vi "FPGA_DAC_move.vi"   [LabVIEW 2010]
uses:
  <vilib>/rvi/DataTransferAndStorage/Container/XNode/niFpgaContainer.xnode
  <vilib>/eio/EIONode/EIONode.xnode
  <vilib>/rvi/eio/nirviEIOImplementation/nirviEIOImplementation.xnode
  <vilib>/rvi/eio/common/nirviEmuClasses.ctl
  <vilib>/rvi/FIFO/Fifo_Resource/nirvififoEmulationSetSize.vi
  <vilib>/rvi/DataTransferAndStorage/Container/Common/niFpgaContainerGetUniqueNameForEmu.vi
  <vilib>/rvi/eio/common/nirviEmuTemplateMethod_noerrors.vi
types:
  T1 = typedef "nirviEmuClasses.ctl" = enum16{"IO Read", "IO Write", "Method", "Property Read", "Property Write"}
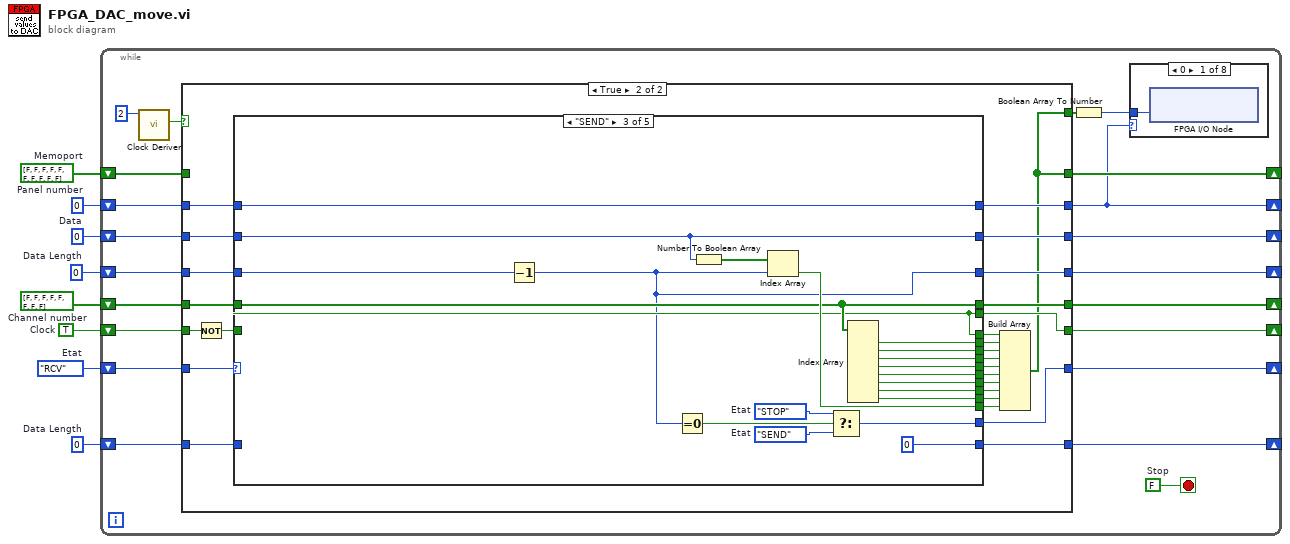
[diagram p0: block diagram]
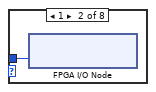
[diagram p2: hidden frame]
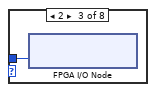
[diagram p3: hidden frame]
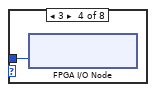
[diagram p4: hidden frame]
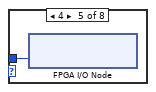
[diagram p5: hidden frame]
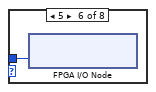
[diagram p6: hidden frame]
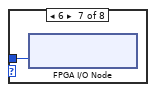
[diagram p7: hidden frame]
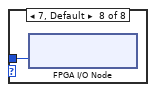
[diagram p8: hidden frame]
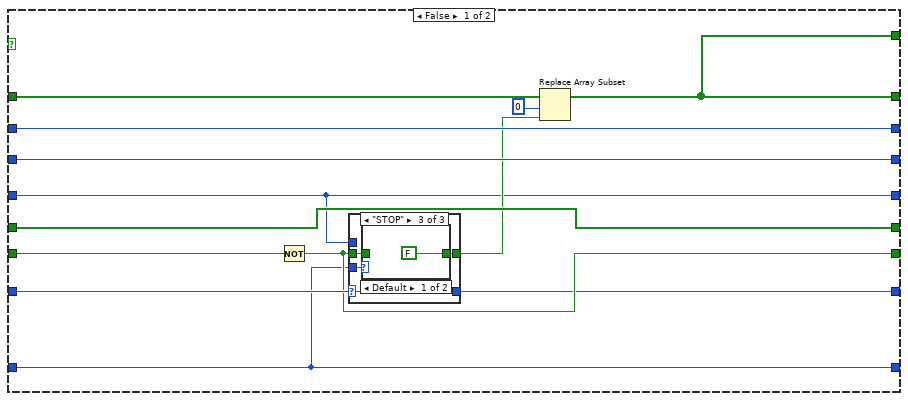
[diagram p9: hidden frame]
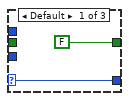
[diagram p10: hidden frame]
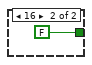
[diagram p12: hidden frame]
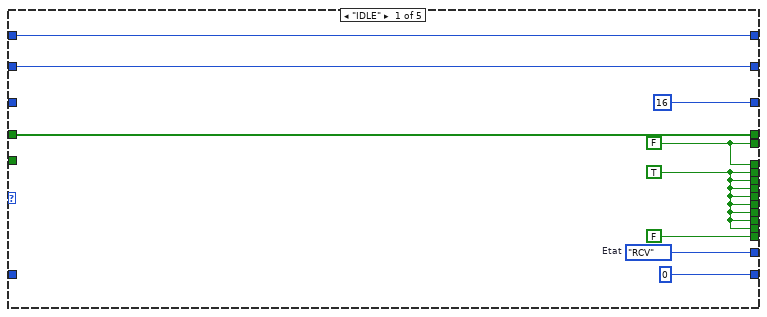
[diagram p14: hidden frame]
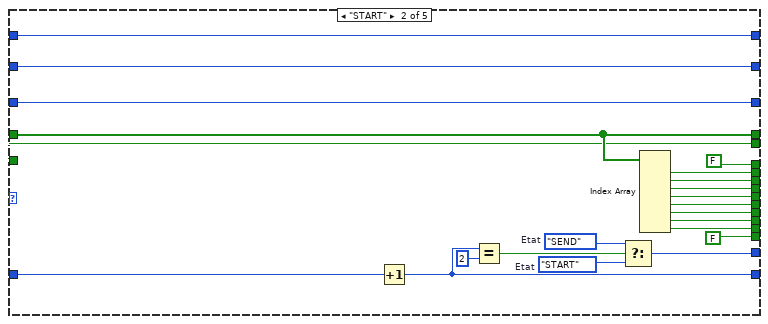
[diagram p15: hidden frame]
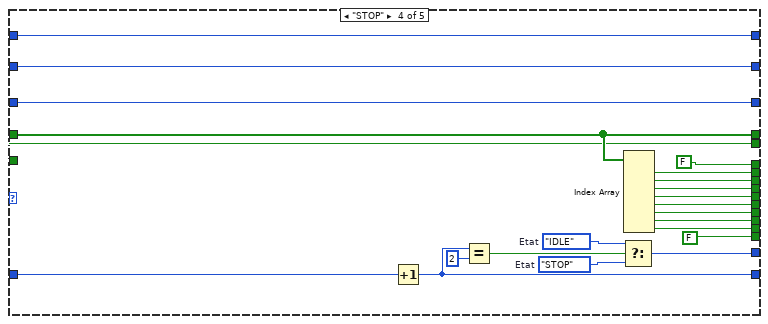
[diagram p16: hidden frame]
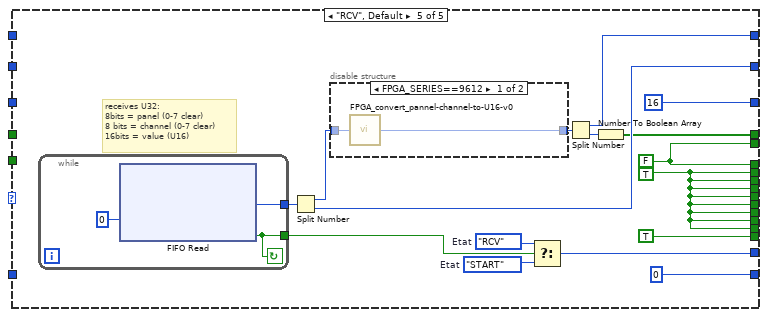
[diagram p17: hidden frame]
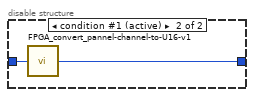
[diagram p18: hidden frame]
diagram:
  w1 = enum8{"IDLE", "START", "SEND", "STOP", "RCV"}."RCV"  # Etat
  w8 = u8 0  # Panel number
  w7 = bool[] [FALSE, FALSE, FALSE, FALSE, FALSE, FALSE, FALSE, FALSE]  # Channel number
  w6 = bool[] [FALSE, FALSE, FALSE, FALSE, FALSE, FALSE, FALSE, FALSE, FALSE, FALSE]  # Memoport
  w5 = u8 0  # Data Length
  w4 = 0  # Data Length
  w3 = u16 0  # Data
  w2 = TRUE  # Clock
  n1 = while {
    shift-right: [w23] -> _
    shift-left: w2 -> [w20]
    shift-right: [w29] -> _
    shift-left: w1 -> [w10]
    shift-right: [w28] -> _
    shift-left: w3 -> [w25]
    shift-right: [w27] -> _
    shift-left: w4 -> [w26]
    shift-right: [w22] -> _
    shift-left: w5 -> [w24]
    shift-right: [w19] -> _
    shift-left: w6 -> [w18]
    shift-right: [w17] -> _
    shift-left: w7 -> [w16]
    shift-right: [w13] -> _
    shift-left: w8 -> [w14]
    stop <- w9 stop-if-true
    w9 = FALSE  # Stop
    n2 = call "Clock Deriver.vi"("Divisor"=u32 2) -> ("Clock Out"=w21:bool)  [unwired: 1 in, 9 out]
    n3 = case shown="True" w21 {
      tunnel: w10 -> [w131 w178]
      tunnel: [w126 w177] -> w29
      tunnel: [w138 w176] -> w28
      tunnel: [w127 w175] -> w27
      tunnel: w26 -> [w127 w174]
      tunnel: w25 -> [w138 w173]
      tunnel: w20 -> [w134 w157]
      tunnel: w24 -> [w128 w172]
      tunnel: [w130 w156] -> w23
      tunnel: [w128 w171] -> w22
      tunnel: [w132 w154] -> w19
      tunnel: w18 -> [w137 _]
      tunnel: [w135 w162] -> w17
      tunnel: w16 -> [w135 w161]
      tunnel: [w133 w159] -> w13
      tunnel: w14 -> [w133 w160]
      tunnel: [w132 w154] -> w11
      frame False {
        n4 = Not(x=w134) -> (.not. x?=w130:bool)
        n5 = case shown="\"STOP\"" w131 {
          selector: w131 -> [w139 w141 w147]
          tunnel: w130 -> [_ w144 w149]
          tunnel: [FALSE w143 w148] -> w129
          tunnel: w128 -> [_ _ w150]
          tunnel: w127 -> [_ w142 _]
          tunnel: [w139 w141 w147] -> w126
          frame Default {
          }
          frame "SEND" {
            n6 = case shown="Default" w142 {
              tunnel: w144 -> [w145 _]
              tunnel: [w145 FALSE] -> w143
              frame Default {
              }
              frame 16 {
              }
            }
          }
          frame "STOP" {
            n7 = case shown="Default" w150 {
              tunnel: w149 -> [_ w152]
              tunnel: [FALSE w152] -> w148
              frame Default {
              }
              frame 0 {
              }
            }
          }
        }
        n8 = Replace Array Subset(array=w137, new element=w129, index=0) -> (w132:bool[])
      }
      frame True {
        n9 = Not(x=w157) -> (.not. x?=w155:bool)
        n10 = case shown="\"SEND\"" w178 {
          tunnel: [w180 w205 w225 w248 w263] -> w177
          tunnel: [w185 w202 w222 w245 w268] -> w164
          tunnel: [w185 w201 w221 w244 w268] -> w165
          tunnel: [w185 w200 w220 w243 w268] -> w166
          tunnel: [w185 w198 w218 w241 w268] -> w168
          tunnel: [w185 w197 w217 w240 w268] -> w169
          tunnel: [w185 w196 w216 w239 w268] -> w170
          tunnel: [FALSE ("CS") FALSE ("CS") w229 FALSE ("CS") TRUE ("CS")] -> w158
          tunnel: [w185 w199 w219 w242 w268] -> w167
          tunnel: [w181 w209 w227 w251 w265] -> w176
          tunnel: [16 ("Data Length") w208 w212 w250 16 ("Data Length")] -> w175
          tunnel: w174 -> [_ w208 w228 w250 _]
          tunnel: w173 -> [w181 w209 w227 w251 _]
          tunnel: w155 -> [_ w193 w213 w236 _]
          tunnel: w172 -> [_ w204 _ w249 _]
          tunnel: [w179 w193 w213 w236 w253] -> w156
          tunnel: [u8 0 ("Data Length") w189 u8 0 ("Data Length") w232 u8 0 ("Data Length")] -> w171
          tunnel: [w185 w203 w223 w246 w268] -> w163
          tunnel: [w183 w195 w215 w238 w264] -> w162
          tunnel: w161 -> [w183 w195 w215 w238 _]
          tunnel: [w182 w194 w214 w237 w255] -> w159
          tunnel: w160 -> [w182 w194 w214 w237 _]
          tunnel: [w179 FALSE w213 FALSE w253] -> w153
          frame "IDLE" {
            w180 = enum8{"IDLE", "START", "SEND", "STOP", "RCV"}."RCV"  # Etat
            w179 = FALSE
            w185 = TRUE ("CS")
          }
          frame "START" {
            w190 = enum8{"IDLE", "START", "SEND", "STOP", "RCV"}."START"  # Etat
            w191 = enum8{"IDLE", "START", "SEND", "STOP", "RCV"}."SEND"  # Etat
            n11 = Increment(x=w204) -> (x+1=w189:u8)
            n12 = Equal?(x=w189, y=u8 2) -> (x = y?=w206:bool)
            n13 = Select(t=w191, s=w206, f=w190) -> (s? t:f=w205:enum8{"IDLE", "START", "SEND", "STOP", "RCV"})
            n14 = Index Array(array=w195) -> (element #1=w203:bool, element #2=w202:bool, element #3=w201:bool, element #4=w200:bool, element #5=w199:bool, element #6=w198:bool, element #7=w197:bool, element #8=w196:bool)  [unwired: 8 in]
          }
          frame "SEND" {
            w210 = enum8{"IDLE", "START", "SEND", "STOP", "RCV"}."SEND"  # Etat
            w211 = enum8{"IDLE", "START", "SEND", "STOP", "RCV"}."STOP"  # Etat
            n15 = Decrement(x=w228) -> (x-1=w212:i32)
            n16 = Equal To 0?(x=w212) -> (x = 0?=w226:bool)
            n17 = Number To Boolean Array(number=w227) -> (Boolean array=w230:bool[])
            n18 = Index Array(array=w230, index=w212) -> (element=w229:bool)
            n19 = Select(t=w211, s=w226, f=w210) -> (s? t:f=w225:enum8{"IDLE", "START", "SEND", "STOP", "RCV"})
            n20 = Index Array(array=w215) -> (element #1=w223:bool, element #2=w222:bool, element #3=w221:bool, element #4=w220:bool, element #5=w219:bool, element #6=w218:bool, element #7=w217:bool, element #8=w216:bool)  [unwired: 8 in]
          }
          frame "STOP" {
            w233 = enum8{"IDLE", "START", "SEND", "STOP", "RCV"}."STOP"  # Etat
            w234 = enum8{"IDLE", "START", "SEND", "STOP", "RCV"}."IDLE"  # Etat
            n21 = Increment(x=w249) -> (x+1=w232:u8)
            n22 = Equal?(x=w232, y=u8 2) -> (x = y?=w247:bool)
            n23 = Select(t=w234, s=w247, f=w233) -> (s? t:f=w248:enum8{"IDLE", "START", "SEND", "STOP", "RCV"})
            n24 = Index Array(array=w238) -> (element #1=w246:bool, element #2=w245:bool, element #3=w244:bool, element #4=w243:bool, element #5=w242:bool, element #6=w241:bool, element #7=w240:bool, element #8=w239:bool)  [unwired: 8 in]
          }
          frame "RCV", Default {
            w258 = enum8{"IDLE", "START", "SEND", "STOP", "RCV"}."RCV"  # Etat
            w259 = enum8{"IDLE", "START", "SEND", "STOP", "RCV"}."START"  # Etat
            w253 = FALSE
            w268 = TRUE ("CS")
            # "receives U32:\n8bits = panel (0-7 clear)\n8 bits = channel (0-7 clear)\n16bits = value (U16)"
            n25 = while {
              tunnel: [w271] -> w261
              tunnel: [w269] -> w260
              stop <- w269 continue-if-true
              n26 = xnode ("FIFO Read")("Timeout"=0) -> ("Element"=w271:u32, "Timed Out?"=w269:bool)  [unwired: 1 in, 1 out]
            }
            n27 = Split Number(x=w261) -> (hi(x)=w257:u16, lo(x)=w265:u16)
            n28 = disable-structure shown="FPGA_SERIES==9612" {
              disable-tunnel: [w324 w325] -> w256
              disable-tunnel: w257 -> [w323 w326]
              frame condition #0 {
                n29 = call "FPGA_convert_pannel-channel-to-U16-v0.vi"("pannel|channel"=w323) -> ("Numérique"=w324:u16)
              }
              frame condition #1 (active) {
                n30 = call "FPGA_convert_pannel-channel-to-U16-v1.vi"("pannel|channel"=w326) -> ("Numérique"=w325:u16)
              }
            }
            n31 = Select(t=w258, s=w260, f=w259) -> (s? t:f=w263:enum8{"IDLE", "START", "SEND", "STOP", "RCV"})
            n32 = Split Number(x=w256) -> (hi(x)=w255:u8, lo(x)=w254:u8)
            n33 = Number To Boolean Array(number=w254) -> (Boolean array=w264:bool[])
          }
        }
        n34 = Build Array(w153, w163, w164, w165, w166, w167, w168, w169, w170, w158) -> (w154:bool[])
      }
    }
    n35 = Boolean Array To Number(Boolean array=w11) -> (number=w12:u16)
    n36 = case shown="0" w13 {
      tunnel: w12 -> [w30 w42 w54 w66 w78 w90 w102 w114]
      frame 0 {
        n37 = xnode "FPGA I/O Node"("Port0/DIO9:0"=w30) -> ()  [unwired: 1 in, 1 out]
      }
      frame 1 {
        n38 = xnode "FPGA I/O Node"("Port1/DIO9:0"=w42) -> ()  [unwired: 1 in, 1 out]
      }
      frame 2 {
        n39 = xnode "FPGA I/O Node"("Port2/DIO9:0"=w54) -> ()  [unwired: 1 in, 1 out]
      }
      frame 3 {
        n40 = xnode "FPGA I/O Node"("Port3/DIO9:0"=w66) -> ()  [unwired: 1 in, 1 out]
      }
      frame 4 {
        n41 = xnode "FPGA I/O Node"("Port4/DIO9:0"=w78) -> ()  [unwired: 1 in, 1 out]
      }
      frame 5 {
        n42 = xnode "FPGA I/O Node"("Port5/DIO9:0"=w90) -> ()  [unwired: 1 in, 1 out]
      }
      frame 6 {
        n43 = xnode "FPGA I/O Node"("Port6/DIO9:0"=w102) -> ()  [unwired: 1 in, 1 out]
      }
      frame 7, Default {
        n44 = xnode "FPGA I/O Node"("Port7/DIO9:0"=w114) -> ()  [unwired: 1 in, 1 out]
      }
    }
  }
